vi "ppanel_plot_hydra_counts.vi"(8 "error in (no error)":errorcluster, 10 "count_rates":T1, 11 "hydraharp_panel in":refnum<class "picoharp_panel.lvclass">) -> (0 "error out":errorcluster, 3 "hydraharp_panel out":refnum<class "picoharp_panel.lvclass">)   [LabVIEW 2015, in "picoharp_panel.lvclass"]
uses:
  picoharp_panel.lvclass
  Hydraharp/hydraharp/hydraharp_count_rates.ctl
  UI/panel_class/panel.lvclass/panel.ctl
  picoharp_panel.lvclass/picoharp_panel.ctl
  UI/panel_class/panel.lvclass
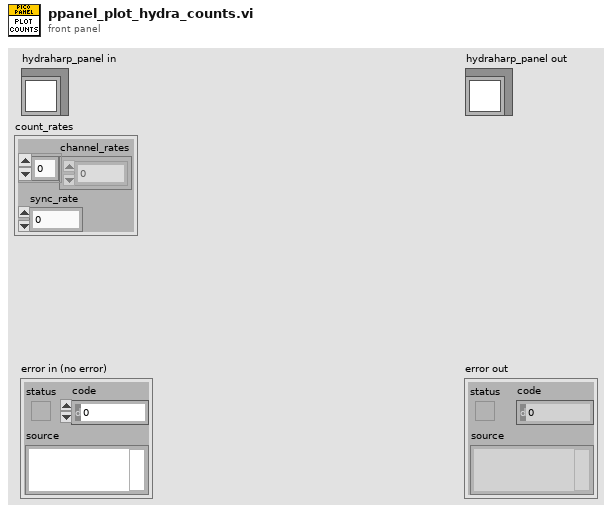
[diagram p1: front panel]
types:
  T1 = typedef "hydraharp_count_rates.ctl" = cluster{"channel_rates":i32[], "sync_rate":i32}
  T2 = typedef "ui_user_events.ctl" = cluster{"update_xy_graph":refnum<user-event>, "update_graph":refnum<user-event>, "update_chart":refnum<user-event>, "update_map":refnum<user-event>, "event_loop_stop":refnum<user-event>, "keep_map":refnum<user-event>}
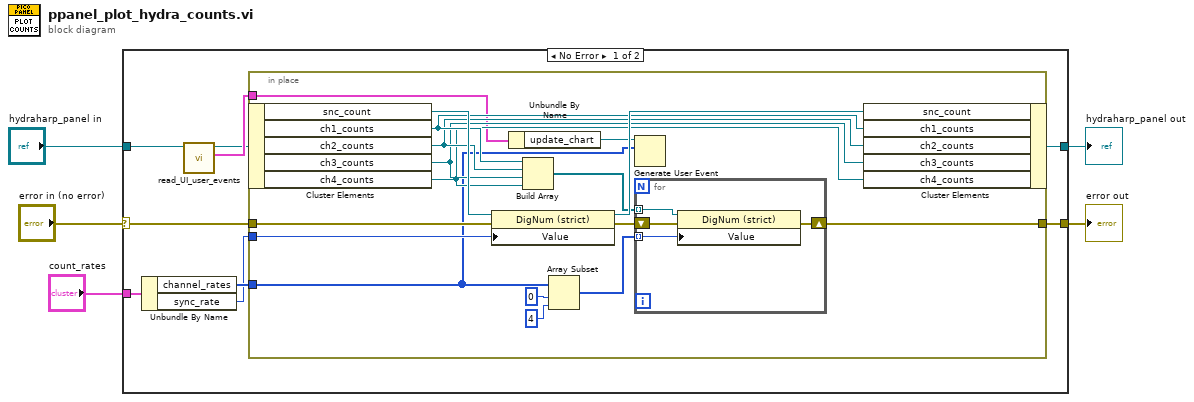
[diagram p0: block diagram]
diagram:
  n1 = case shown="No Error" "error in (no error)" {
    selector: "error in (no error)" -> [w10 w37]
    tunnel: [w9 w37] -> w4
    tunnel: [w12 w36] -> w2
    tunnel: "hydraharp_panel in" -> [w8 w36]
    tunnel: "count_rates" -> [w14 _]
    frame No Error {
      n2 = Unbundle By Name(w14) -> ("channel_rates"=w13:i32[], "sync_rate"=w11:i32)
      n3 = call "read_UI_user_events.vi"("panel in"=w8) -> ("ui_user_events"=w7:T2, "panel out"=w6:refnum<class "picoharp_panel.lvclass">)  [unwired: 8 in, 1 out]
      n4 = in-place {
        in-place-border: w13 -> [w16]
        in-place-border: w11 -> [w28]
        in-place-border: w10 -> [w26]
        in-place-border: [w23] -> w9
        in-place-border: w7 -> [w18]
        n5 = in-place-cluster #1(w6) -> ("snc_count"=w29:refnum<vi>, "ch1_counts"=w22:refnum<vi>, "ch2_counts"=w21:refnum<vi>, "ch3_counts"=w20:refnum<vi>, "ch4_counts"=w19:refnum<vi>)
        n6 = property class="DigNum (strict)"(reference=w29, error in=w26, "Value"=w28) -> (reference out=w27:refnum<vi>, error out=w15:errorcluster)
        n7 = Unbundle By Name(w18) -> ("update_chart"=w17:refnum<user-event>)
        n8 = Build Array(w22, w21, w20, w19) -> (w24:refnum<vi>[])
        n9 = Array Subset(array=w16, index=0, length=4) -> (w25:i32[])
        n10 = Generate User Event(user event=w17, event data cluster=w16) -> ()  [unwired: 2 in, 2 out]
        n11 = for {
          tunnel: w25 -> [w35] mode=indexing
          shift-right: [w32] -> w23
          shift-left: w15 -> [w33]
          tunnel: w24 -> [w34] mode=indexing
          n12 = property class="DigNum (strict)"(reference=w34, error in=w33, "Value"=w35) -> (error out=w32:errorcluster)  [unwired: 1 out]
        }
        n13 = in-place-cluster #1("snc_count"=w27, "ch1_counts"=w22, "ch2_counts"=w21, "ch3_counts"=w20, "ch4_counts"=w19) -> (w12:refnum<class "picoharp_panel.lvclass">)
      }
    }
    frame Error {
    }
  }
  "error out" <- w4
  "hydraharp_panel out" <- w2
